vi "Read(Impedance).vi"(8 "error in (no error)":errorcluster, 11 "VISA resource name":refnum<visa-resource-name>) -> (0 "error out":errorcluster, 2 "Comparator Result":string, 3 "VISA resource name out":refnum<visa-resource-name>, 4 "Monitor2 Value":dbl, 5 "Secondary Value":dbl, 6 "Monitor1 Value":dbl, 7 "Primary Value":dbl)   [LabVIEW 2021, in "LCR Meter.lvlib"]
doc: "Query the latest measurement data of the primary parameter, secondary parameter, monitor1 and monitor2 results into the output buffer."
uses:
  LCR Meter.lvlib
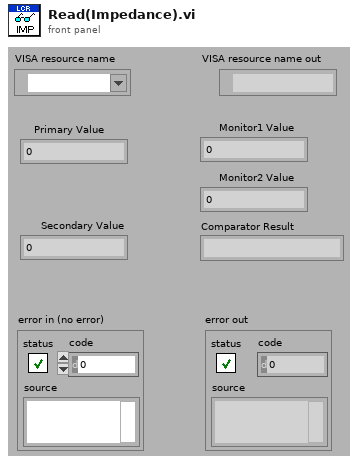
[diagram p1: front panel]
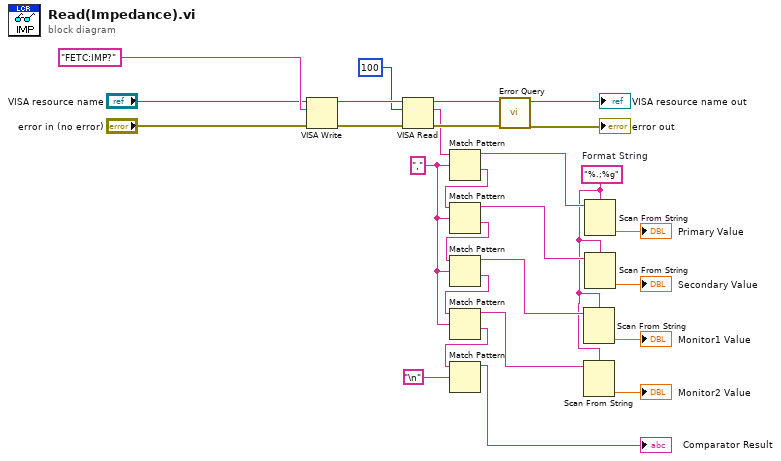
[diagram p0: block diagram]
diagram:
  w3 = "%.;%g"  # Format String
  w9 = "," ("regular expression")
  n1 = VISA Write(VISA resource name="VISA resource name", write buffer="FETC:IMP?", error in (no error)="error in (no error)") -> (VISA resource name out=w22:refnum<visa-resource-name>, error out=w21:errorcluster)  [unwired: 1 out]
  n2 = VISA Read(VISA resource name=w22, byte count=u32 100, error in (no error)=w21) -> (VISA resource name out=w20:refnum<visa-resource-name>, read buffer=w1:string, error out=w19:errorcluster)  [unwired: 1 out]
  n3 = Match Pattern(string=w1, regular expression=w9) -> (before substring=w15:string, after substring=w10:string)  [unwired: 1 in, 2 out]
  n4 = Match Pattern(string=w10, regular expression=w9) -> (before substring=w14:string, after substring=w13:string)  [unwired: 1 in, 2 out]
  n5 = Match Pattern(string=w13, regular expression=w9) -> (before substring=w5:string, after substring=w12:string)  [unwired: 1 in, 2 out]
  n6 = Match Pattern(string=w12, regular expression=w9) -> (before substring=w4:string, after substring=w11:string)  [unwired: 1 in, 2 out]
  n7 = Match Pattern(string=w11, regular expression="\n") -> (before substring=→"Comparator Result":string)  [unwired: 1 in, 3 out]
  n8 = call "Error Query.vi"("error in (no error)"=w19, "VISA resource name"=w20) -> ("error out"=→"error out":errorcluster, "VISA resource name out"=→"VISA resource name out":refnum<visa-resource-name>)  [unwired: 6 in, 2 out]
  n9 = Scan From String(format string=w3, input string=w5) -> (output 1=→"Monitor1 Value":dbl)  [unwired: 3 in, 3 out]
  n10 = Scan From String(format string=w3, input string=w4) -> (output 1=→"Monitor2 Value":dbl)  [unwired: 3 in, 3 out]
  n11 = Scan From String(format string=w3, input string=w15) -> (output 1=→"Primary Value":dbl)  [unwired: 3 in, 3 out]
  n12 = Scan From String(format string=w3, input string=w14) -> (output 1=→"Secondary Value":dbl)  [unwired: 3 in, 3 out]
